vi "_Read.vi"(8 "error in (no error)":errorcluster, 9 "Timeout S (0)":dbl, 10 "Bytes to Read (0)":i32, 11 "VisaResource in":refnum<class "VisaResource.lvclass">) -> (0 "error out":errorcluster, 1 "Bytes Read":i32, 2 "Data":string, 3 "VisaResource out":refnum<class "VisaResource.lvclass">)   [LabVIEW 2020, in "PicoG-Core.lvlib" / "VisaResource.lvclass"]
doc: "<b>Bytes to Read</b>:\n -1 to read as many bytes as possible until timeout\n 0 to return current bytes available immediately, ignoring timeout.\n >0 to wait for number of bytes until timeout"
uses:
  VisaResource.lvclass
  VisaResource.lvclass/VisaResource.ctl
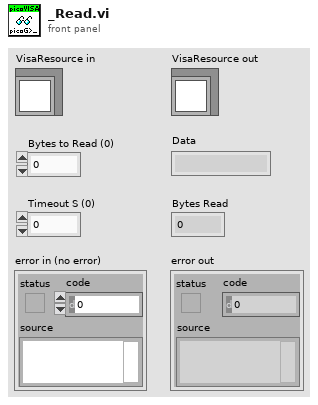
[diagram p1: front panel]
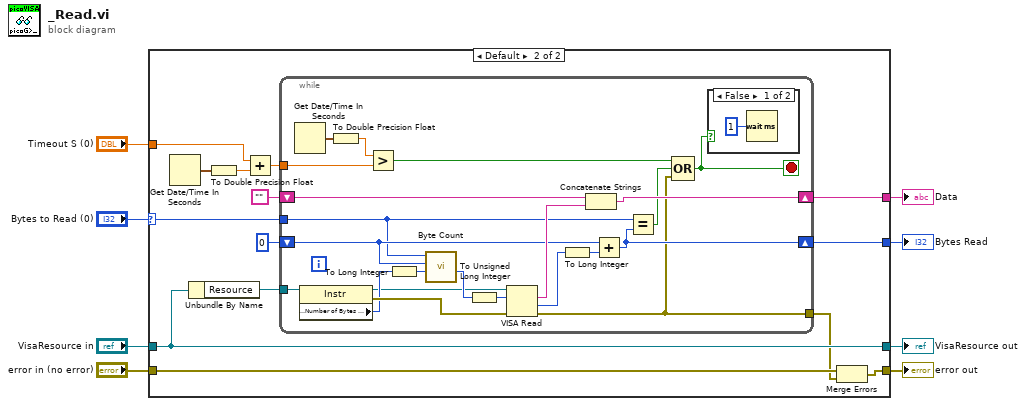
[diagram p0: block diagram]
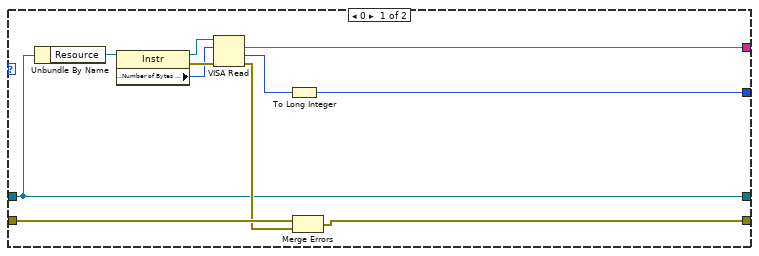
[diagram p2: hidden frame]
diagram:
  n1 = case shown="Default" "Bytes to Read (0)" {
    selector: "Bytes to Read (0)" -> [_ w30]
    tunnel: "Timeout S (0)" -> [_ w31]
    tunnel: "VisaResource in" -> [w10 w25]
    tunnel: "error in (no error)" -> [w13 w28]
    tunnel: [w15 w21] -> w4
    tunnel: [w9 w26] -> w3
    tunnel: [w11 w27] -> w2
    tunnel: [w10 w25] -> w1
    frame 0 {
      n2 = Unbundle By Name(w10) -> ("Resource"=w18:refnum<visa-resource-name>)
      n3 = property class="Instr"(reference=w18) -> (reference out=w16:refnum<visa-resource-name>, error out=w19:errorcluster, "Serial Settings:Number of Bytes at Serial Port"=w17:u32)  [unwired: 1 in]
      n4 = VISA Read(VISA resource name=w16, byte count=w17, error in (no error)=w19) -> (read buffer=w15:string, return count=w14:u32, error out=w12:errorcluster)  [unwired: 1 out]
      n5 = To Long Integer(number=w14) -> (32bit integer=w9:i32)
      n6 = Merge Errors(w13, w12) -> (w11:errorcluster)
    }
    frame Default {
      n7 = Get Date/Time In Seconds() -> (seconds since 1Jan1904=w33:timestamp)
      n8 = Unbundle By Name(w25) -> ("Resource"=w24:refnum<visa-resource-name>)
      n9 = To Double Precision Float(number=w33) -> (double precision float=w32:dbl)
      n10 = Add(x=w31, y=w32) -> (x+y=w23:dbl)
      n11 = while {
        tunnel: w30 -> [w42]
        shift-right: [w43] -> w26
        shift-left: 0 -> [w45]
        tunnel: w24 -> [w51]
        tunnel: w23 -> [w53]
        shift-right: [w47] -> w21
        shift-left: "" -> [w48]
        tunnel: [w39] -> w20
        stop <- w35 stop-if-true
        n12 = Get Date/Time In Seconds() -> (seconds since 1Jan1904=w54:timestamp)
        n13 = property class="Instr"(reference=w51) -> (reference out=w34:refnum<visa-resource-name>, error out=w55:errorcluster, "Serial Settings:Number of Bytes at Serial Port"=w50:u32)  [unwired: 1 in]
        n14 = To Double Precision Float(number=w54) -> (double precision float=w52:dbl)
        n15 = Greater?(x=w52, y=w53) -> (0:w41:bool)
        n16 = To Long Integer(number=w50) -> (32bit integer=w37:i32)
        n17 = call "Byte Count.vi"("Bytes Available"=w37, "Bytes so far"=w45, "Bytes to Read"=w42) -> ("Byte count"=w49:i32)  [unwired: 8 in]
        n18 = To Unsigned Long Integer(number=w49) -> (unsigned 32bit integer=w36:u32)
        n19 = VISA Read(VISA resource name=w34, byte count=w36, error in (no error)=w55) -> (read buffer=w46:string, return count=w44:u32, error out=w39:errorcluster)  [unwired: 1 out]
        n20 = To Long Integer(number=w44) -> (32bit integer=w38:i32)
        n21 = Concatenate Strings(w48, w46) -> (w47:string)
        n22 = Add(x=w45, y=w38) -> (x+y=w43:i32)
        n23 = Equal?(x=w42, y=w43) -> (x = y?=w40:bool)
        n24 = Compound Arithmetic op=OR(w41, w40, w39) -> (w35:bool)
        n25 = case shown="False" w35 {
          frame False {
            n26 = Wait (ms)(milliseconds to wait=u32 1) -> ()  [unwired: 1 out]
          }
          frame True {
          }
        }
      }
      n27 = Merge Errors(w28, w20) -> (w27:errorcluster)
    }
  }
  "error out" <- w2
  "VisaResource out" <- w1
  "Bytes Read" <- w3
  "Data" <- w4
